vi "MouseoverList.vi"(8 "error in (no error)":errorcluster, 10 "Click Details":T1, 11 "UI Refs":T2) -> (0 "error out":errorcluster)   [LabVIEW 2015]
uses:
  Controls & Type Defs/UI Data.ctl
  Controls & Type Defs/ClickDetails.ctl
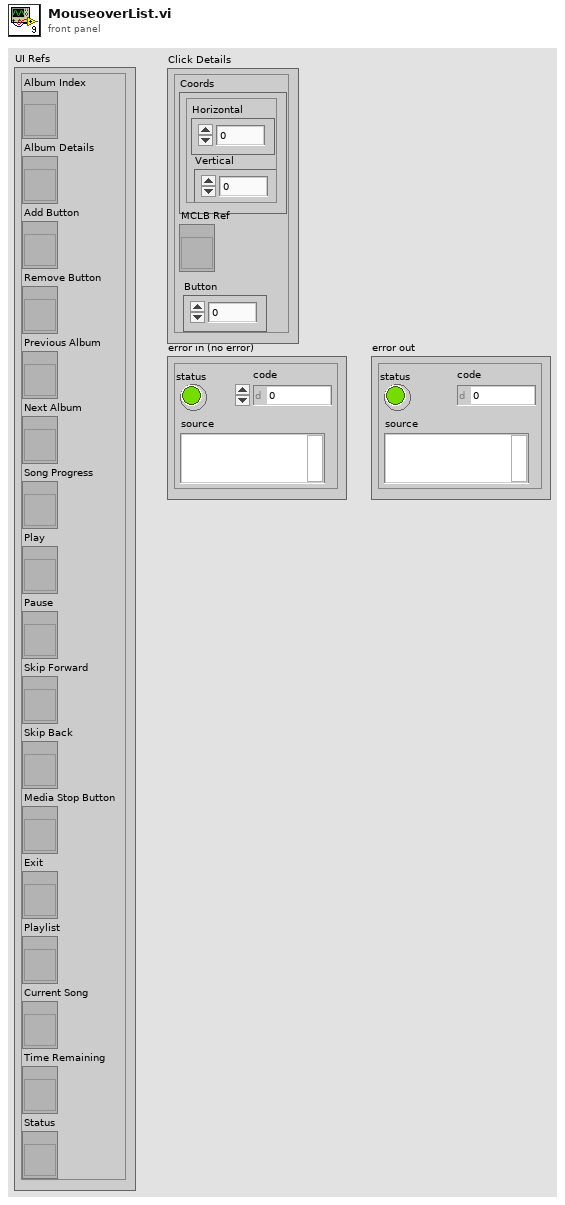
[diagram p1: front panel]
types:
  T1 = typedef "ClickDetails.ctl" = cluster{"Coords":cluster{"Vertical":i32, "Horizontal":i32}, "MCLB Ref":refnum<vi>, "Button":u16}
  T2 = typedef "UI Data.ctl" = cluster{"Album Index":refnum<vi>, "Album Details":refnum<vi>, "Add Button":refnum<vi>, "Remove Button":refnum<vi>, "Previous Album":refnum<vi>, "Next Album":refnum<vi>, "Song Progress":refnum<vi>, "Play":refnum<vi>, "Pause ":refnum<vi>, "Skip Forward":refnum<vi>, "Skip Back":refnum<vi>, "Media Stop Button":refnum<vi>, "Exit":refnum<vi>, "Playlist":refnum<vi>, "Current Song":refnum<vi>, "Time Remaining":refnum<vi>, "Status":refnum<vi>}
  T3 = typedef "LVRowAndColumnTypeDef.ctl" = cluster{"Row":i32, "Column":i32}
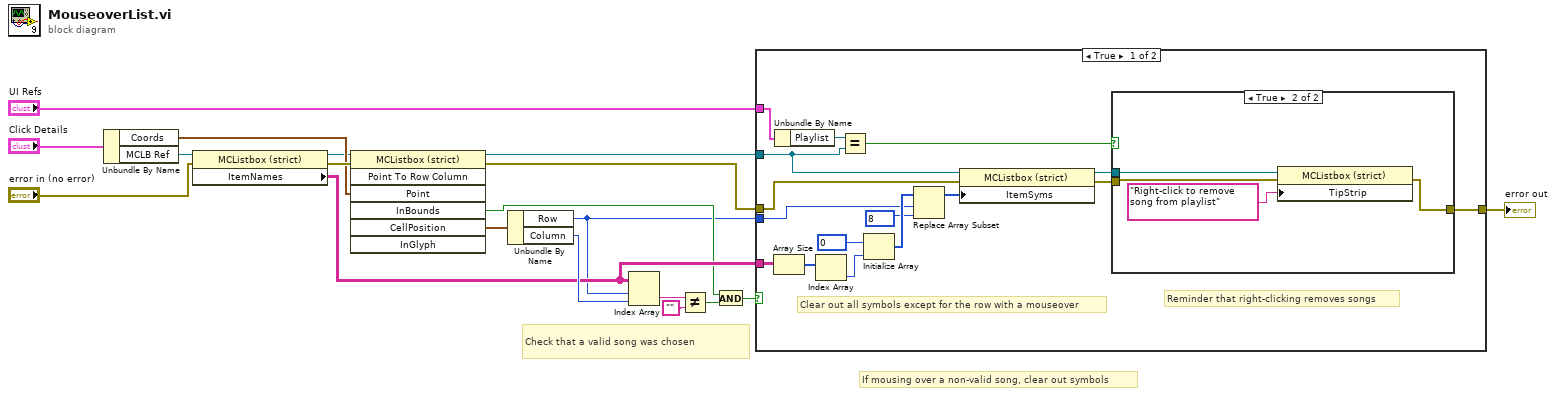
[diagram p0: block diagram]
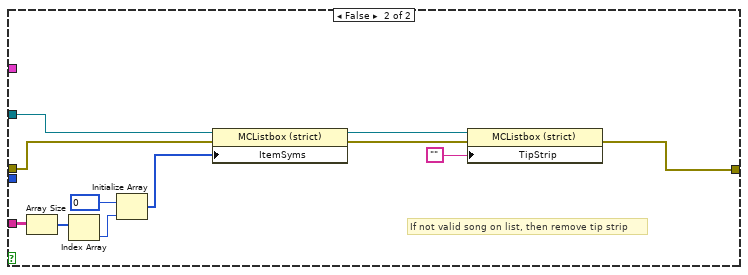
[diagram p3: hidden frame]
diagram:
  # "If mousing over a non-valid song, clear out symbols"
  # "Check that a valid song was chosen"
  n1 = Unbundle By Name("Click Details") -> ("Coords"=w18:cluster{"Vertical":i32, "Horizontal":i32}, "MCLB Ref"=w4:refnum<vi>)
  n2 = property class="MCListbox (strict)"(reference=w4, error in="error in (no error)") -> (reference out=w3:refnum<vi>, error out=w19:errorcluster, "ItemNames"=w11:string[][])
  n3 = invoke class="MCListbox (strict)" method="Point To Row Column"(reference=w3, error in=w19, "Point"=w18) -> (reference out=w2:refnum<vi>, error out=w12:errorcluster, "InBounds"=w8:bool, "CellPosition"=w15:T3)  [unwired: 4 in, 3 out]
  n4 = Unbundle By Name(w15) -> ("Row"=w1:i32, "Column"=w16:i32)
  n5 = Index Array(array=w11, index (row)=w1, index (col)=w16) -> (element=w14:string)
  n6 = Not Equal?(x=w14, y="") -> (x != y?=w7:bool)
  n7 = And(x=w8, y=w7) -> (x .and. y?=w6:bool)
  n8 = case shown="True" w6 {
    tunnel: "UI Refs" -> [w35 _]
    tunnel: w12 -> [w23 w46]
    tunnel: w11 -> [w31 w50]
    tunnel: [w21 w41] -> w10
    tunnel: w2 -> [w32 w51]
    tunnel: w1 -> [w24 _]
    frame True {
      # "Reminder that right-clicking removes songs"
      # "Clear out all symbols except for the row with a mouseover"
      n9 = Array Size(array=w31) -> (size(s)=w30:i32[])
      n10 = Unbundle By Name(w35) -> ("Playlist"=w34:refnum<vi>)
      n11 = Index Array(array=w30) -> (element=w29:i32)  [unwired: 1 in]
      n12 = Equal?(x=w34, y=w32) -> (x = y?=w33:bool)
      n13 = Initialize Array(0, w29) -> (w26:i32[])
      n14 = Replace Array Subset(array=w26, new element=8, index=w24) -> (w27:i32[])
      n15 = property class="MCListbox (strict)"(reference=w32, error in=w23, "ItemSyms"=w27) -> (reference out=w20:refnum<vi>, error out=w22:errorcluster)
      n16 = case shown="True" w33 {
        tunnel: w22 -> [w36 w40]
        tunnel: [w36 w37] -> w21
        tunnel: w20 -> [_ w39]
        frame False {
        }
        frame True {
          n17 = property class="MCListbox (strict)"(reference=w39, error in=w40, "TipStrip"="Right-click to remove song from playlist" ("Tip Strip")) -> (error out=w37:errorcluster)  [unwired: 1 out]
        }
      }
    }
    frame False {
      # "If not valid song on list, then remove tip strip"
      n18 = Array Size(array=w50) -> (size(s)=w49:i32[])
      n19 = Index Array(array=w49) -> (element=w48:i32)  [unwired: 1 in]
      n20 = Initialize Array(0, w48) -> (w45:i32[])
      n21 = property class="MCListbox (strict)"(reference=w51, error in=w46, "ItemSyms"=w45) -> (reference out=w44:refnum<vi>, error out=w43:errorcluster)
      n22 = property class="MCListbox (strict)"(reference=w44, error in=w43, "TipStrip"="") -> (error out=w41:errorcluster)  [unwired: 1 out]
    }
  }
  "error out" <- w10
